vi "SlewRateLimiter_Execute.vi"(9 "Enable":bool=TRUE, 10 "Rate":dbl, 11 "Input":dbl) -> (1 "Output":dbl, 3 "out SLEW_RATE_LIMITER":T1 {"PrevTime" format="%30.5p"; "PrevValue" format="%13.5p"; "RateLimit" format="%13.5p"})   [LabVIEW 2019, in "Trajectory_Library.lvlib"]
doc: "Convience, single call, LabVIEW function. Creates and calculates the slew rate limiter function to filter the input to limit its slew rate. The optional enable parameter bypasses the filter calculation when \"enabled\" is false. When enabled is \"false\" the input is passed directly to the output and the internal buffer is continually filled with the current input value.\n\n\nThis limits the rate of change of an input value. Useful for implementing voltage, setpoint, and/or output ramps. A slew-rate limit is most appropriate when the quantity being controlled is a velocity or a voltage; when controlling a position, consider using a postion control algoritmn or trapezoid profile instead.\n\nInputs:\n - input -- The input value whose slew rate is to be limited.\n - rate -- The new rate limit in units/second.\n - enable -- Perform the rate limit calcuation when True. When False, output the input value unchanged. (Default=True)\n\nOutputs:\n - out Slew Rate Limiter -- The modified Slew Rate Limiter data cluster\n - output -- The filtered value, which will not change faster than the slew rate."
uses:
  Trajectory_Library.lvlib
  SLEW_RATE_LIMITER.ctl
  Util_GetTime.vi
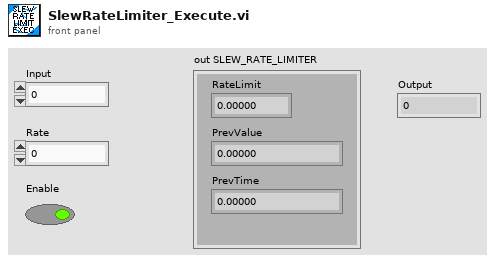
[diagram p1: front panel]
types:
  T1 = typedef "Trajectory_Library.lvlib/SLEW_RATE_LIMITER.ctl" = cluster{"RateLimit":dbl, "PrevValue":dbl, "PrevTime":dbl}
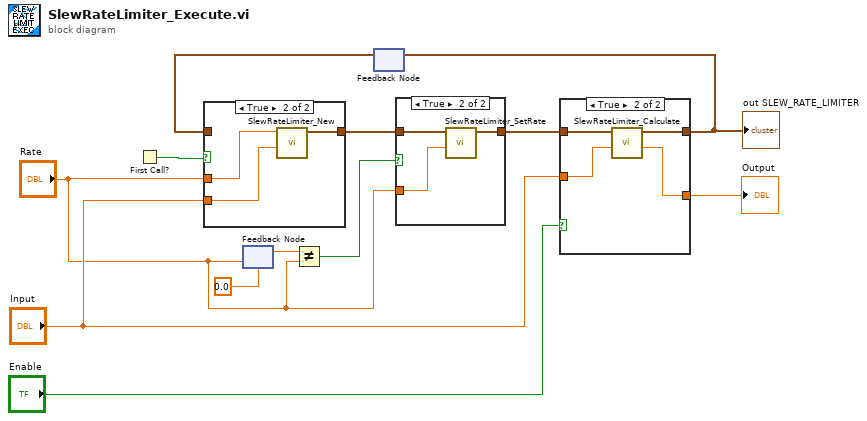
[diagram p0: block diagram]
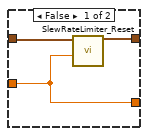
[diagram p3: hidden frame]
diagram:
  n1 = First Call?() -> (First Call?: T/F=w11:bool)
  n2 = feedback #1(0.0 ("Rate")) -> (w5:dbl)
  n3 = feedback-in #1("Rate") -> ()
  n4 = Not Equal?(x=w5, y="Rate") -> (x != y?=w2:bool)
  n5 = feedback #2() -> (w12:T1)  [unwired: 1 in]
  n6 = case shown="True" w11 {
    tunnel: [w13 w16] -> w6
    tunnel: w12 -> [w13 _]
    tunnel: "Rate" -> [_ w15]
    tunnel: "Input" -> [_ w14]
    frame False {
    }
    frame True {
      n7 = call "SlewRateLimiter_New.vi"("InitialValue"=w14, "RateLimit"=w15) -> ("out SLEW_RATE_LIMITER"=w16:T1)  [unwired: 9 in]
    }
  }
  n8 = case shown="True" w2 {
    tunnel: w6 -> [w17 w19]
    tunnel: [w17 w20] -> w1
    tunnel: "Rate" -> [_ w18]
    frame False {
    }
    frame True {
      n9 = call "SlewRateLimiter_SetRate.vi"("Rate"=w18, "in SLEW_RATE_LIMITER"=w19) -> ("out SLEW_RATE_LIMITER"=w20:T1)  [unwired: 9 in]
    }
  }
  n10 = case shown="True" "Enable" {
    tunnel: w1 -> [w23 w27]
    tunnel: [w21 w26] -> w10
    tunnel: [w22 w25] -> w9
    tunnel: "Input" -> [w22 w24]
    frame False {
      n11 = call "SlewRateLimiter_Reset.vi"("ResetValue"=w22, "in SLEW_RATE_LIMITER"=w23) -> ("out SLEW_RATE_LIMITER"=w21:T1)  [unwired: 9 in]
    }
    frame True {
      n12 = call "SlewRateLimiter_Calculate.vi"("Input"=w24, "in SLEW_RATE_LIMITER"=w27) -> ("Output"=w25:dbl, "out SLEW_RATE_LIMITER"=w26:T1)  [unwired: 8 in]
    }
  }
  "out SLEW_RATE_LIMITER" <- w10
  "Output" <- w9
  n13 = feedback-in #2(w10) -> ()
